vi "ReadProjectFromController_Example.vi"(8 "Fehler (Eingang, kein Fehler)":errorcluster, 11 "ControllerIP":string="192.168.5.24") -> (0 "Fehler (Ausgang)":errorcluster, 3 "ControllerID":string)   [LabVIEW 2016]
uses:
  girpcutil_params.ctl
panel:
  out "ConnectionToken":string
  out "ProjectPath":string
  out "ProjectID":string
  out "State":string
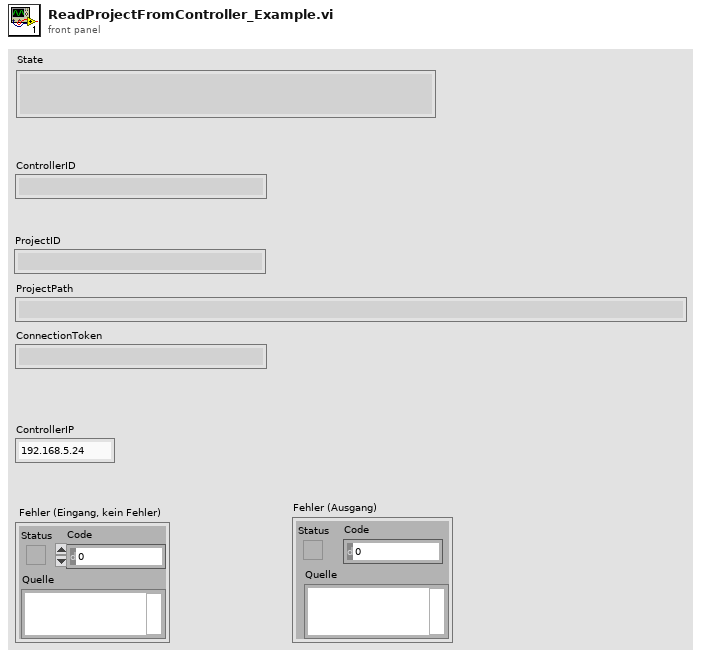
[diagram p1: front panel]
types:
  T1 = typedef "girpcutil_params.ctl" = cluster{"ConnectionHandle":i32, "DLL-Handle":cluster{"DLL Path":path, "Is32Bit":bool}}
  T2 = enum16{"Bool", "Snippet", "Struct", "Int64", "Int32", "Float", "Double", "String"}
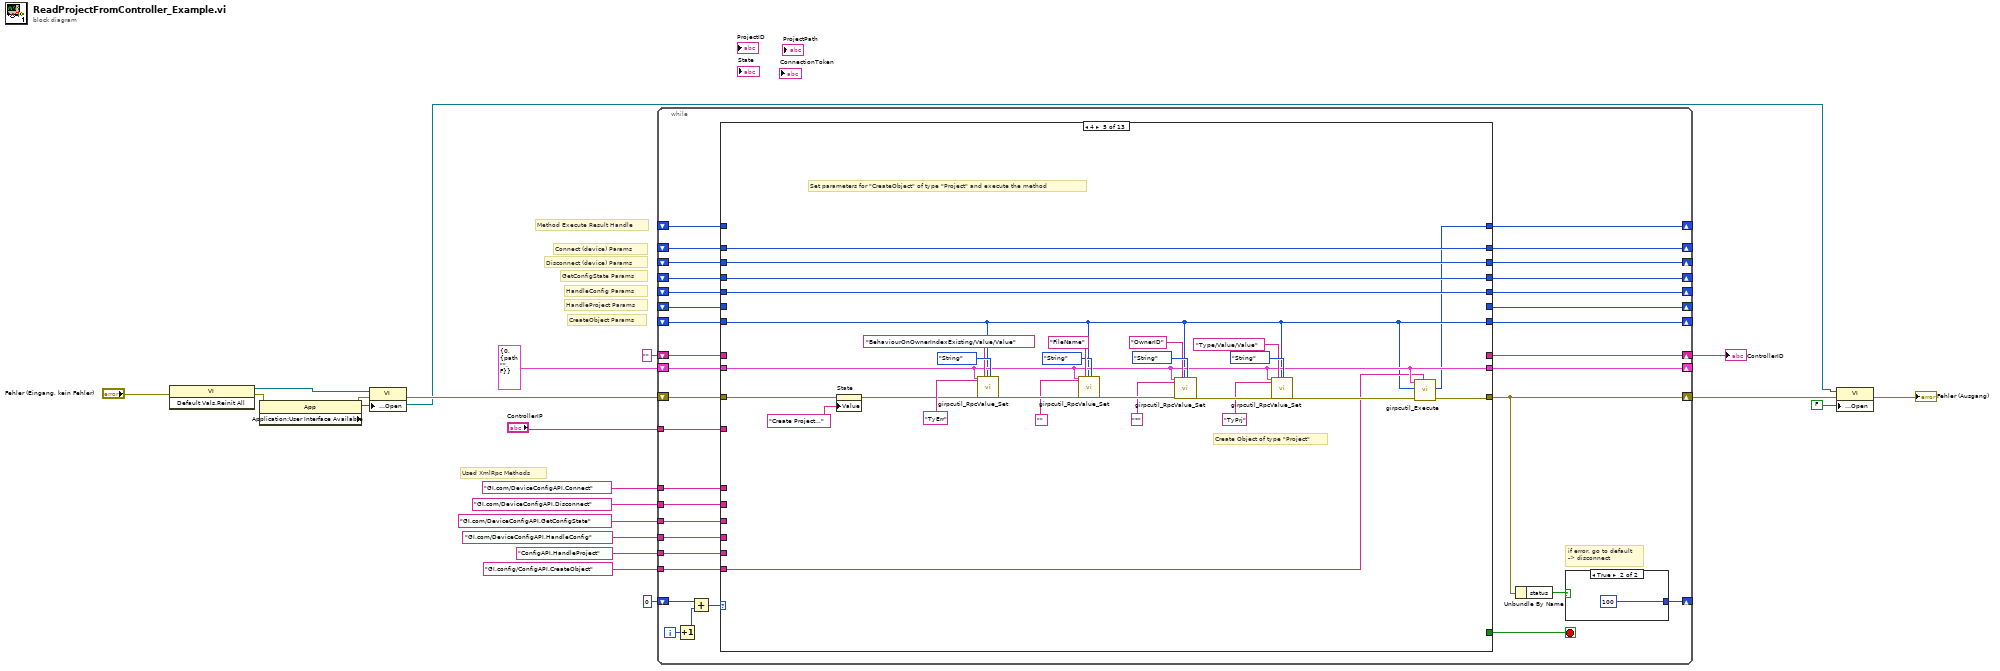
[diagram p0: block diagram]
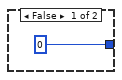
[diagram p2: hidden frame]
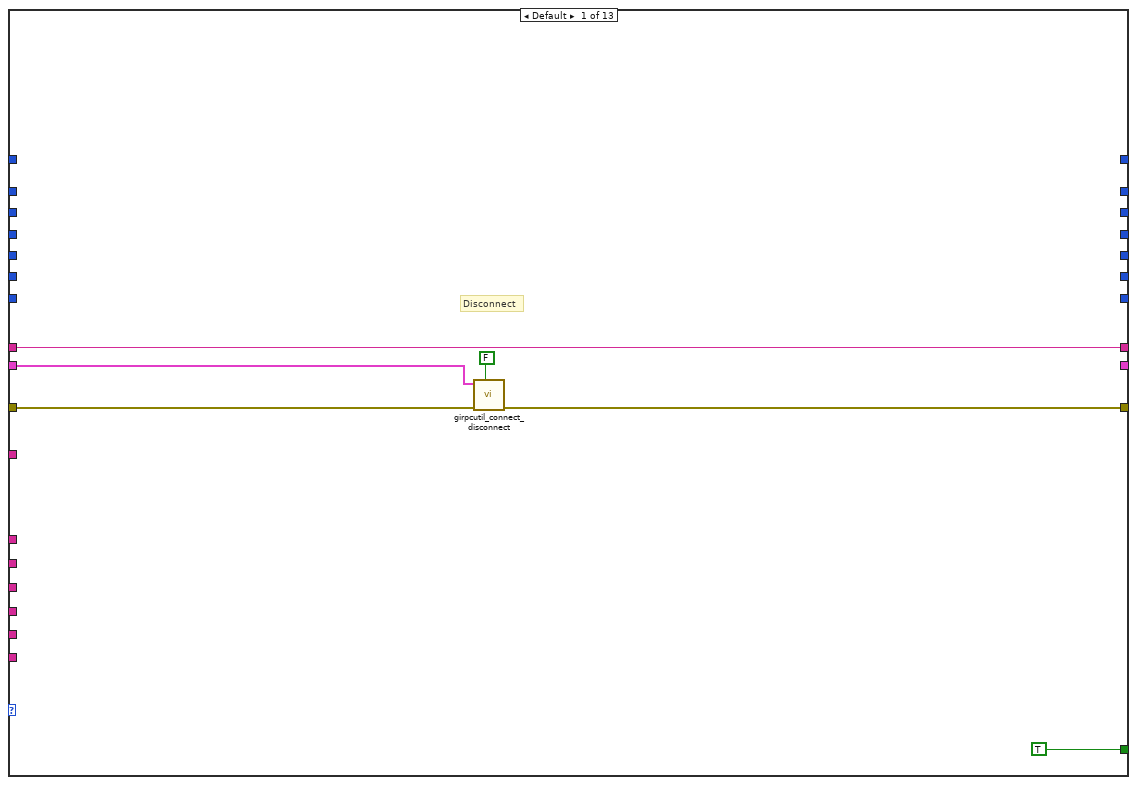
[diagram p3: hidden frame]
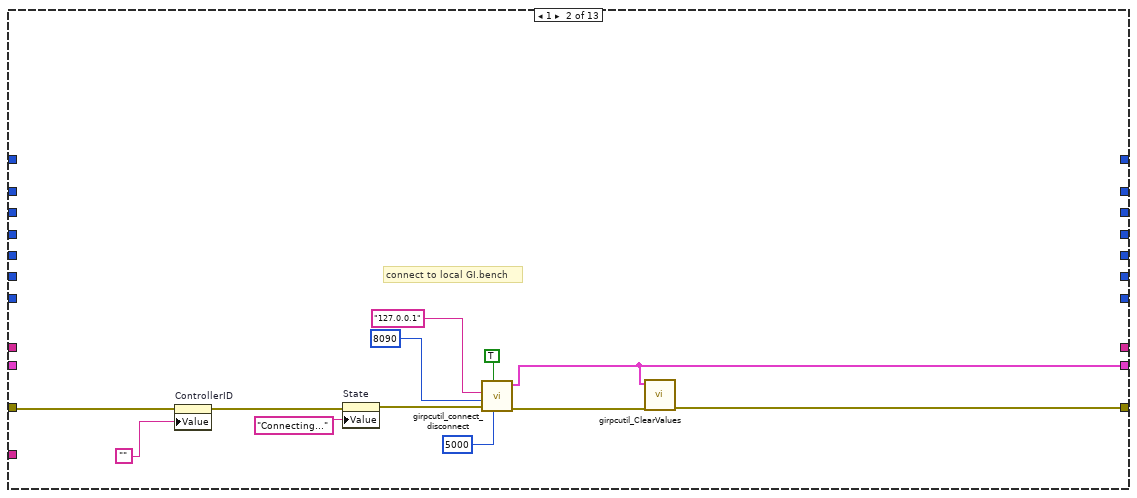
[diagram p4: hidden frame]
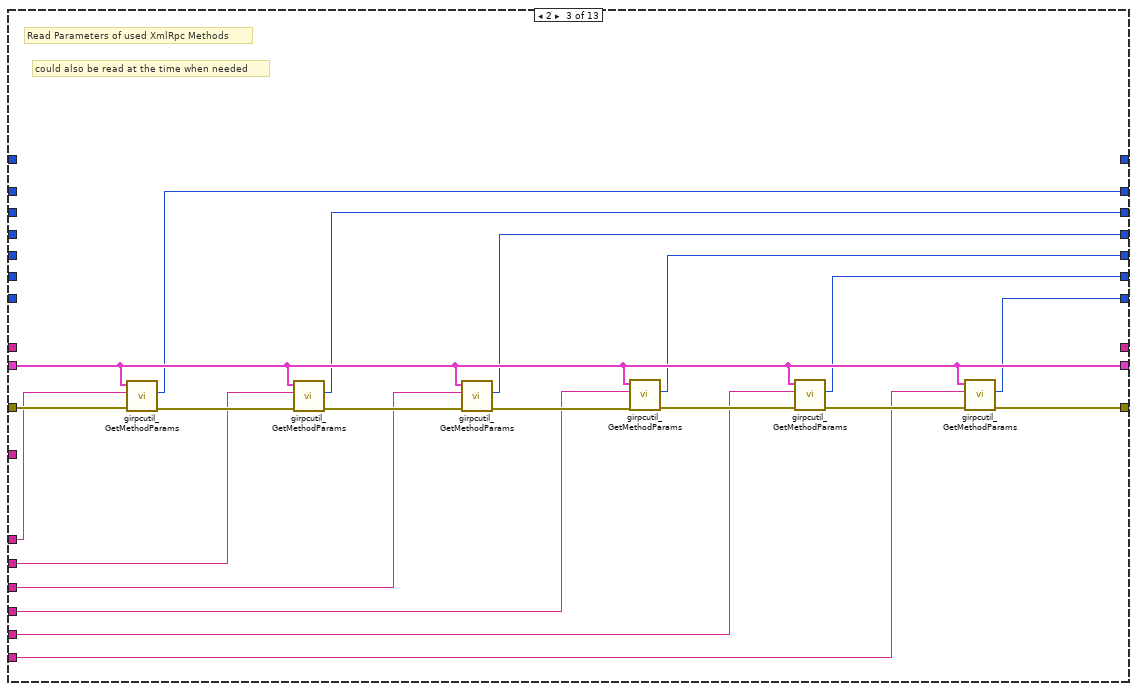
[diagram p5: hidden frame]
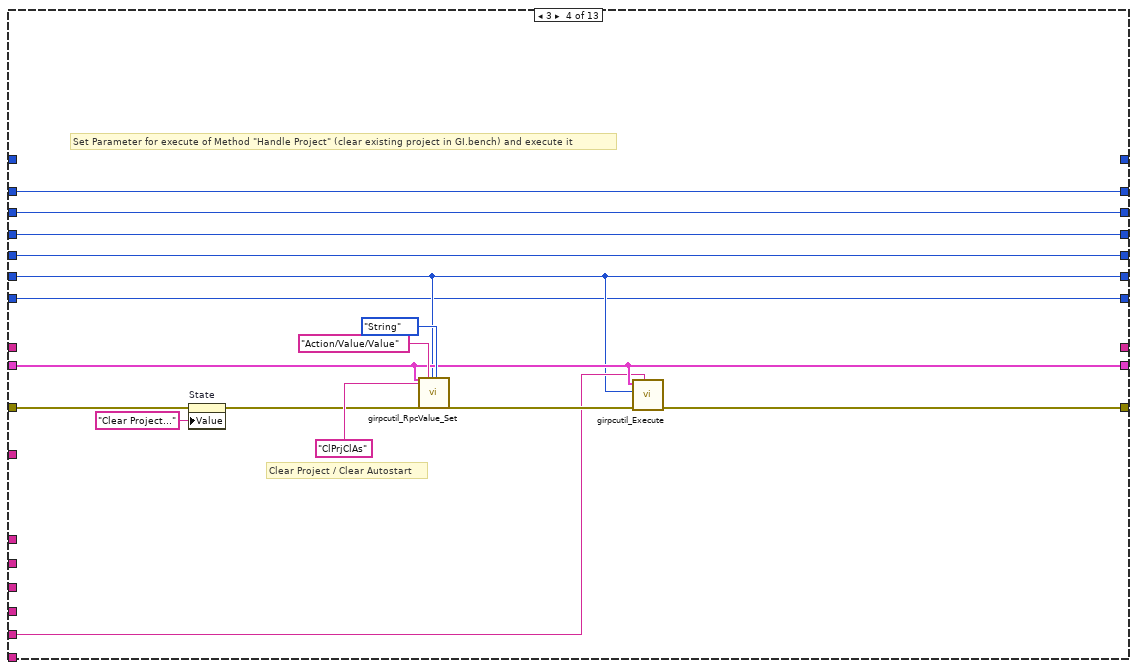
[diagram p6: hidden frame]
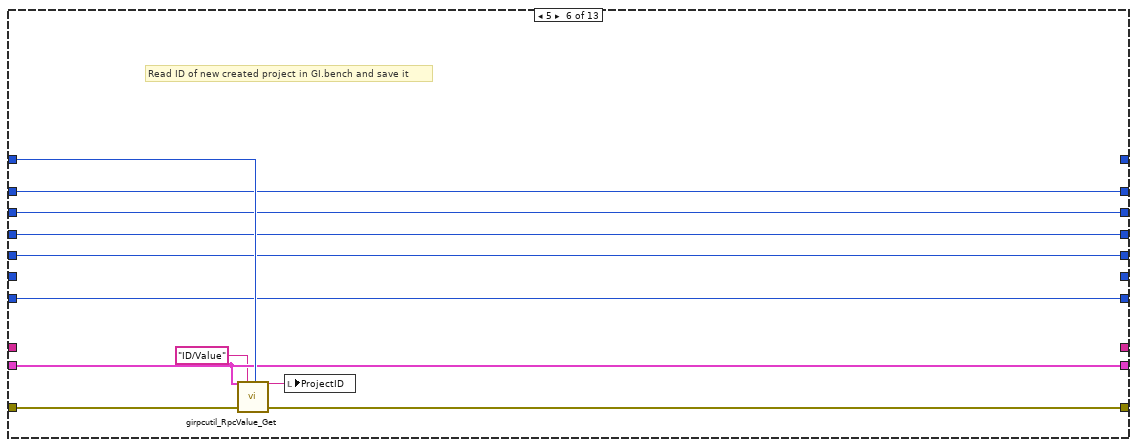
[diagram p7: hidden frame]
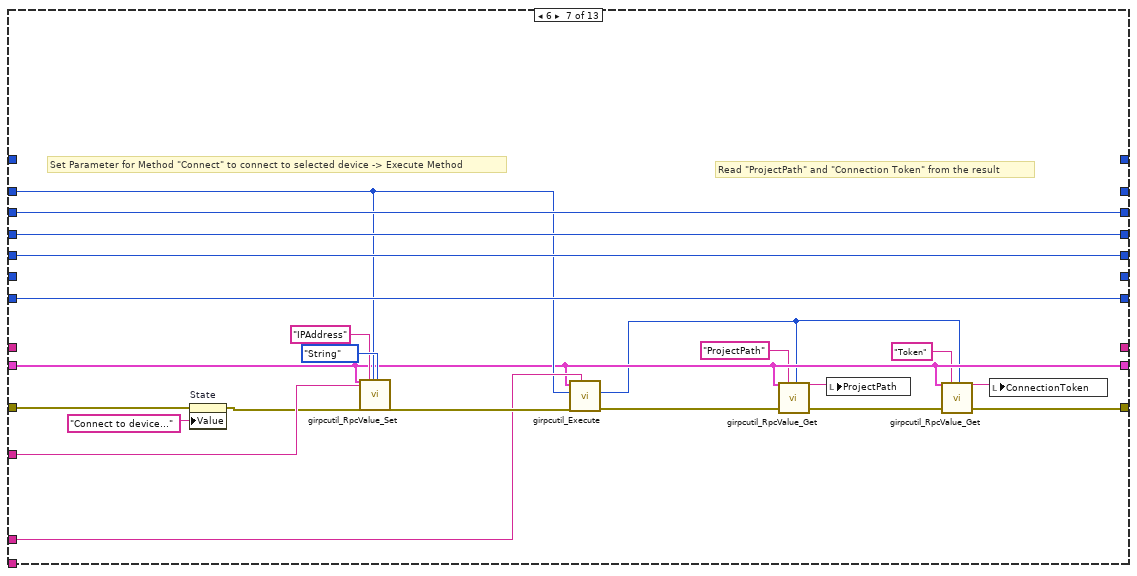
[diagram p8: hidden frame]
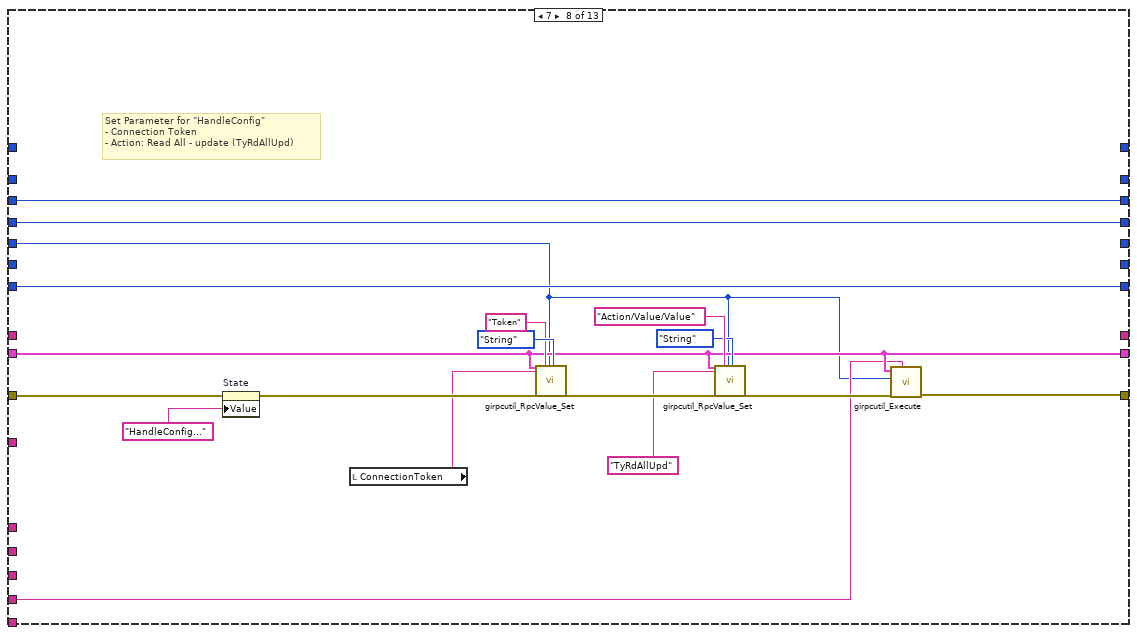
[diagram p9: hidden frame]
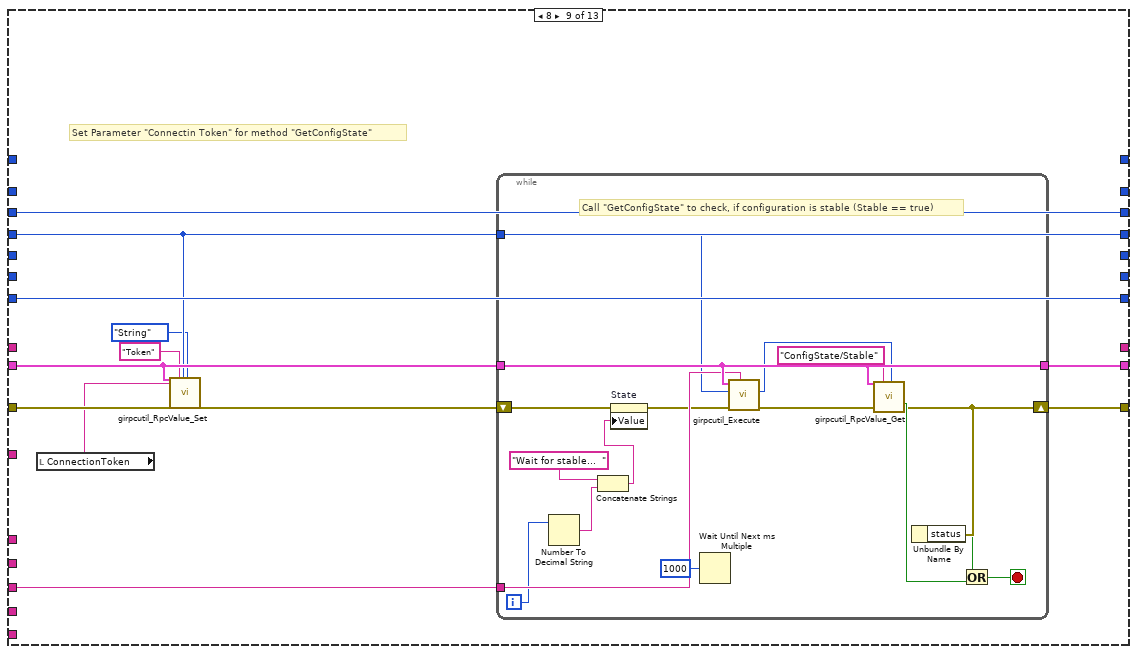
[diagram p10: hidden frame]
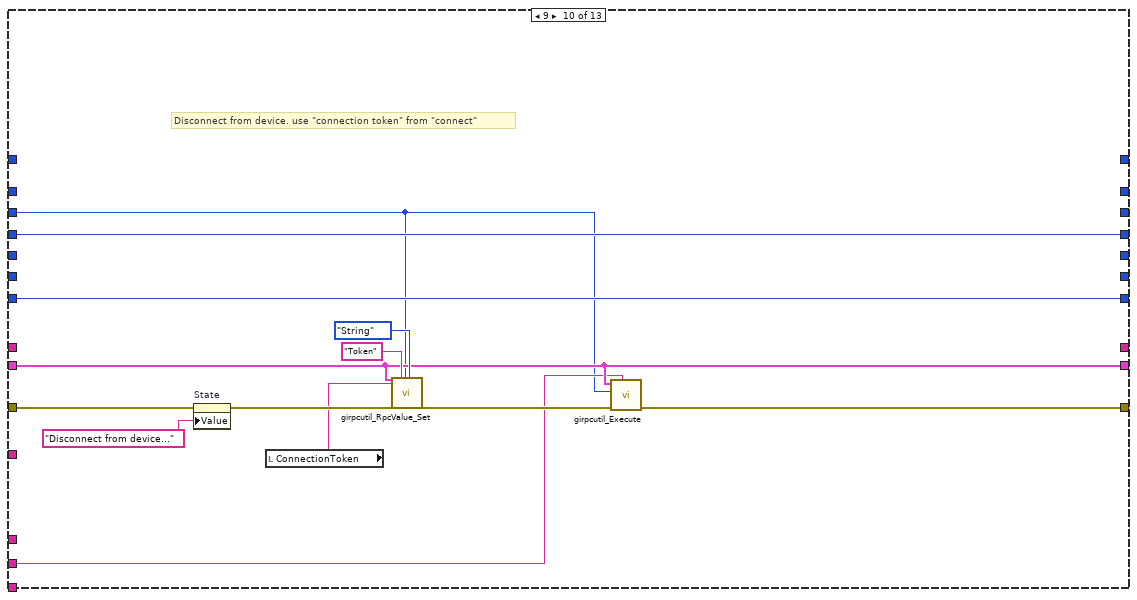
[diagram p11: hidden frame]
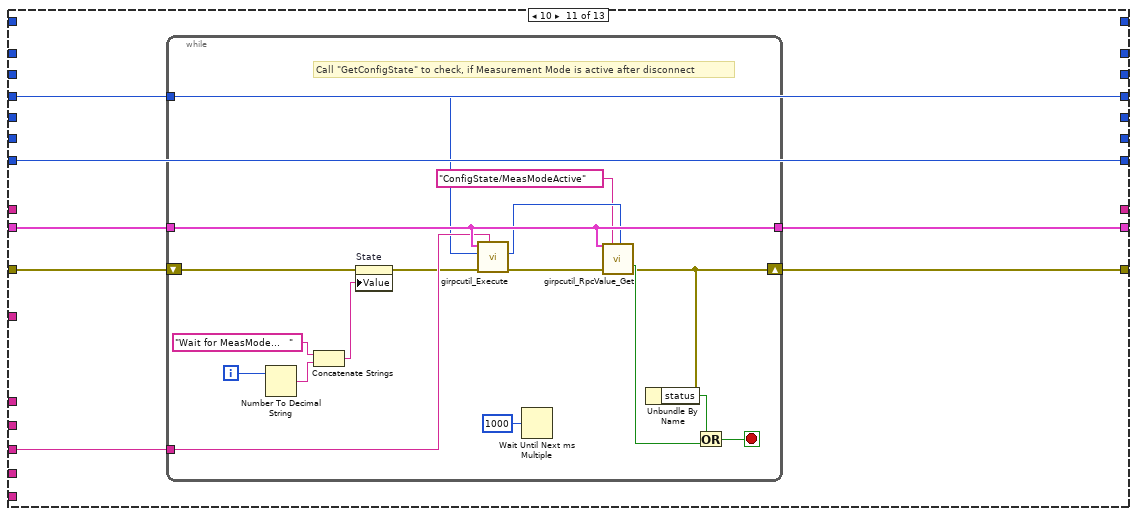
[diagram p12: hidden frame]
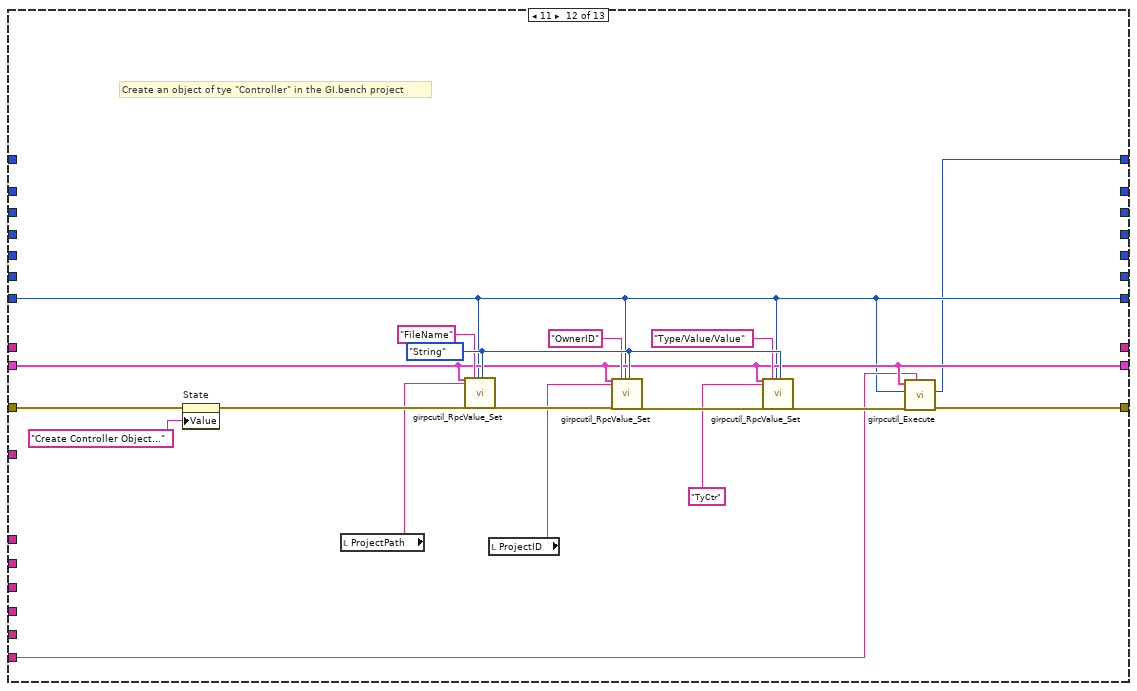
[diagram p13: hidden frame]
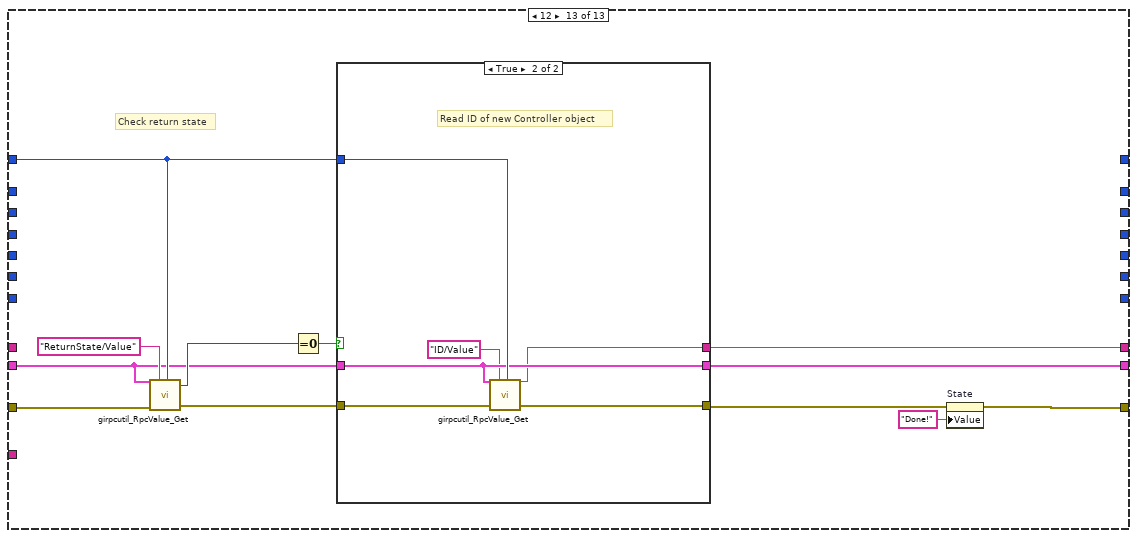
[diagram p14: hidden frame]
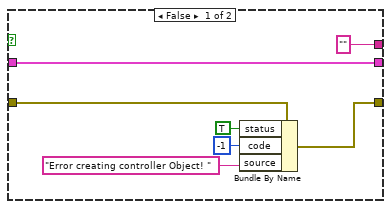
[diagram p15: hidden frame]
diagram:
  # "Method Execute Result Handle"
  # "CreateObject Params"
  # "HandleProject Params"
  # "HandleConfig Params"
  # "GetConfigState Params"
  # "Disconnect (device) Params"
  # "Connect (device) Params"
  # "Used XmlRpc Methods"
  n1 = invoke class="VI" method="Default Vals.Reinit All"(error in="Fehler (Eingang, kein Fehler)") -> (reference out=w13:refnum<vi>, error out=w11:errorcluster)  [unwired: 2 in, 1 out]
  n2 = property class="App"(error in=w11) -> (error out=w10:errorcluster, "Application:User Interface Available"=w12:bool)  [unwired: 1 in, 1 out]
  n3 = property class="VI"(reference=w13, error in=w10, "Front Panel.Open"=w12) -> (reference out=w4:refnum<vi>, error out=w9:errorcluster)
  n4 = while {
    shift-right: [w39] -> w6
    shift-left: w9 -> [w54]
    tunnel: "GI.com/DeviceConfigAPI.Connect" ("methodName") -> [w53]
    tunnel: "GI.com/DeviceConfigAPI.Disconnect" ("methodName") -> [w52]
    tunnel: "GI.com/DeviceConfigAPI.GetConfigState" ("methodName") -> [w51]
    tunnel: "GI.com/DeviceConfigAPI.HandleConfig" ("methodName") -> [w50]
    tunnel: "ConfigAPI.HandleProject" ("methodName") -> [w49]
    tunnel: "GI.config/ConfigAPI.CreateObject" ("methodName") -> [w48]
    shift-right: [w47] -> _
    shift-left: T1 {"ConnectionHandle"=0, "DLL-Handle"={"DLL Path"=path "", "Is32Bit"=FALSE}} ("girpcutil_params 2") -> [w46]
    shift-right: [w45] -> _
    shift-left: _ -> [w37]
    shift-right: [w44] -> _
    shift-left: _ -> [w36]
    shift-right: [w43] -> _
    shift-left: _ -> [w35]
    shift-right: [w42] -> _
    shift-left: _ -> [w34]
    shift-right: [w41] -> _
    shift-left: _ -> [w38]
    shift-right: [w40] -> _
    shift-left: _ -> [w33]
    shift-right: [w32] -> _
    shift-left: _ -> [w31]
    tunnel: "ControllerIP" -> [w30]
    shift-right: [w29] -> w15
    shift-left: "" ("StringResult") -> [w28]
    shift-right: [w22] -> _
    shift-left: 0 -> [w23]
    i -> [w55]
    stop <- w27 stop-if-true
    # "if error, go to default\n-> disconnect"
    n5 = Increment(x=w55) -> (x+1=w25:i32)
    n6 = Add(x=w23, y=w25) -> (x+y=w24:i32)
    n7 = case shown="4" w24 {
      tunnel: [TRUE _ _ _ _ _ _ _ _ _ _ _ _] -> w27
      tunnel: w54 -> [w62 w66 w95 w97 w113 w150 w154 w175 w197 w222 w239 w260 w286]
      tunnel: [w61 w70 w89 w107 w116 w146 w160 w177 w200 w227 w238 w266 w275] -> w39
      tunnel: w53 -> [_ _ w87 _ _ _ w164 _ _ _ _ _ _]
      tunnel: w52 -> [_ _ w86 _ _ _ _ _ _ w228 _ _ _]
      tunnel: w51 -> [_ _ w85 _ _ _ _ _ w201 _ w233 _ _]
      tunnel: w50 -> [_ _ w84 _ _ _ _ w179 _ _ _ _ _]
      tunnel: w49 -> [_ _ w83 w105 _ _ _ _ _ _ _ _ _]
      tunnel: w48 -> [_ _ w82 _ w118 _ _ _ _ _ _ w264 _]
      tunnel: [_ w69 w88 w106 w119 w148 w159 w180 w202 w229 w236 w265 w280] -> w47
      tunnel: w46 -> [w60 _ w88 w106 w119 w148 w159 w180 w195 w229 w237 w265 w279]
      tunnel: [_ _ w81 w103 w139 w145 _ _ _ _ _ _ _] -> w45
      tunnel: [_ _ w80 w102 w138 w144 w172 w188 w199 _ _ _ _] -> w44
      tunnel: [_ _ w79 w101 w137 w143 w171 w187 w194 w225 w235 _ _] -> w43
      tunnel: [_ _ w78 w100 w136 w142 w170 _ _ _ _ _ _] -> w42
      tunnel: [_ _ w77 w104 _ _ _ _ _ _ _ _ _] -> w41
      tunnel: [_ _ w76 w99 w117 w141 w169 w186 w198 w226 w234 w263 _] -> w40
      tunnel: w38 -> [_ _ _ w104 _ _ _ _ _ _ _ _ _]
      tunnel: w37 -> [_ _ _ w103 w139 w145 w163 _ _ _ _ _ _]
      tunnel: w36 -> [_ _ _ w102 w138 w144 w172 w188 w199 w224 _ _ _]
      tunnel: w35 -> [_ _ _ w101 w137 w143 w171 w187 w194 w225 w235 _ _]
      tunnel: w34 -> [_ _ _ w100 w136 w142 w170 w178 _ _ _ _ _]
      tunnel: w33 -> [_ _ _ w99 w117 w141 w169 w186 w198 w226 w234 w263 _]
      tunnel: [_ _ _ _ w115 _ _ _ _ _ _ w262 _] -> w32
      tunnel: w31 -> [_ _ _ _ _ w149 _ _ _ _ _ _ w281]
      tunnel: w30 -> [_ _ _ _ _ _ w166 _ _ _ _ _ _]
      tunnel: [w59 _ _ _ _ _ _ _ _ _ _ _ w278] -> w29
      tunnel: w28 -> [w59 _ _ _ _ _ _ _ _ _ _ _ _]
      frame Default {
        # "Disconnect"
        n8 = call "girpcutil_connect_disconnect.vi"("Connect"=FALSE, "Fehler (Eingang, kein Fehler)"=w62, "girpcutil_params"=w60) -> ("Fehler (Ausgang)"=w61:errorcluster)  [unwired: 7 in, 1 out]
      }
      frame 1 {
        # "connect to local GI.bench"
        n9 = property on="ControllerID" class="Str"(error in=w66, "Value"="") -> (error out=w65:errorcluster)  [unwired: 1 in, 1 out]
        n10 = property on="State" class="Str"(error in=w65, "Value"="Connecting..." ("State")) -> (error out=w68:errorcluster)  [unwired: 1 in, 1 out]
        n11 = call "girpcutil_connect_disconnect.vi"("timeout"=u32 5000, "Connect"=TRUE, "Fehler (Eingang, kein Fehler)"=w68, "port"=u32 8090, "host"="127.0.0.1") -> ("Fehler (Ausgang)"=w71:errorcluster, "girpcutil_params 2"=w69:T1)  [unwired: 5 in]
        n12 = call "girpcutil_ClearValues.vi"("Fehler (Eingang, kein Fehler)"=w71, "girpcutil_params"=w69) -> ("error IO"=w70:errorcluster)  [unwired: 9 in]
      }
      frame 2 {
        # "could also be read at the time when needed"
        # "Read Parameters of used XmlRpc Methods"
        n13 = call "girpcutil_GetMethodParams.vi"("Fehler (Eingang, kein Fehler)"=w95, "methodName"=w87, "girpcutil_params"=w88) -> ("Fehler (Ausgang)"=w94:errorcluster, "param handle out"=w81:i32)  [unwired: 7 in]
        n14 = call "girpcutil_GetMethodParams.vi"("Fehler (Eingang, kein Fehler)"=w94, "methodName"=w86, "girpcutil_params"=w88) -> ("Fehler (Ausgang)"=w93:errorcluster, "param handle out"=w80:i32)  [unwired: 7 in]
        n15 = call "girpcutil_GetMethodParams.vi"("Fehler (Eingang, kein Fehler)"=w93, "methodName"=w85, "girpcutil_params"=w88) -> ("Fehler (Ausgang)"=w92:errorcluster, "param handle out"=w79:i32)  [unwired: 7 in]
        n16 = call "girpcutil_GetMethodParams.vi"("Fehler (Eingang, kein Fehler)"=w92, "methodName"=w84, "girpcutil_params"=w88) -> ("Fehler (Ausgang)"=w91:errorcluster, "param handle out"=w78:i32)  [unwired: 7 in]
        n17 = call "girpcutil_GetMethodParams.vi"("Fehler (Eingang, kein Fehler)"=w91, "methodName"=w83, "girpcutil_params"=w88) -> ("Fehler (Ausgang)"=w90:errorcluster, "param handle out"=w77:i32)  [unwired: 7 in]
        n18 = call "girpcutil_GetMethodParams.vi"("Fehler (Eingang, kein Fehler)"=w90, "methodName"=w82, "girpcutil_params"=w88) -> ("Fehler (Ausgang)"=w89:errorcluster, "param handle out"=w76:i32)  [unwired: 7 in]
      }
      frame 3 {
        # "Clear Project / Clear Autostart"
        # "Set Parameter for execute of Method \"Handle Project\" (clear existing project in GI.bench) and execute it"
        n19 = property on="State" class="Str"(error in=w97, "Value"="Clear Project..." ("State")) -> (error out=w96:errorcluster)  [unwired: 1 in, 1 out]
        n20 = call "girpcutil_RpcValue_Set.vi"("girpcutil_params"=w106, "StringValue or Snippet"="ClPrjClAs", "Fehler (Eingang, kein Fehler)"=w96, "MemberName"="Action/Value/Value", "param handle"=w104, "DataType"=T2."String") -> ("Fehler (Ausgang)"=w108:errorcluster)  [unwired: 21 in]
        n21 = call "girpcutil_Execute.vi"("methodName"=w105, "Fehler (Eingang, kein Fehler)"=w108, "params"=w104, "girpcutil_params"=w106) -> ("Fehler (Ausgang)"=w107:errorcluster)  [unwired: 6 in, 1 out]
      }
      frame 4 {
        # "Create Object of type \"Project\""
        # "Set parameters for \"CreateObject\" of type \"Project\" and execute the method"
        n22 = property on="State" class="Str"(error in=w113, "Value"="Create Project..." ("State")) -> (error out=w112:errorcluster)  [unwired: 1 in, 1 out]
        n23 = call "girpcutil_RpcValue_Set.vi"("girpcutil_params"=w119, "StringValue or Snippet"="TyErr", "Fehler (Eingang, kein Fehler)"=w112, "MemberName"="BehaviourOnOwnerIndexExisting/Value/Value", "param handle"=w117, "DataType"=T2."String") -> ("Fehler (Ausgang)"=w132:errorcluster)  [unwired: 21 in]
        n24 = call "girpcutil_RpcValue_Set.vi"("girpcutil_params"=w119, "StringValue or Snippet"="", "Fehler (Eingang, kein Fehler)"=w132, "MemberName"="FileName", "param handle"=w117, "DataType"=T2."String") -> ("Fehler (Ausgang)"=w128:errorcluster)  [unwired: 21 in]
        n25 = call "girpcutil_RpcValue_Set.vi"("girpcutil_params"=w119, "StringValue or Snippet"="*", "Fehler (Eingang, kein Fehler)"=w128, "MemberName"="OwnerID", "param handle"=w117, "DataType"=T2."String") -> ("Fehler (Ausgang)"=w124:errorcluster)  [unwired: 21 in]
        n26 = call "girpcutil_RpcValue_Set.vi"("girpcutil_params"=w119, "StringValue or Snippet"="TyPrj", "Fehler (Eingang, kein Fehler)"=w124, "MemberName"="Type/Value/Value", "param handle"=w117, "DataType"=T2."String") -> ("Fehler (Ausgang)"=w120:errorcluster)  [unwired: 21 in]
        n27 = call "girpcutil_Execute.vi"("methodName"=w118, "Fehler (Eingang, kein Fehler)"=w120, "params"=w117, "girpcutil_params"=w119) -> ("Fehler (Ausgang)"=w116:errorcluster, "results"=w115:i32)  [unwired: 6 in]
      }
      frame 5 {
        # "Read ID of new created project in GI.bench and save it"
        n28 = call "girpcutil_RpcValue_Get.vi"("girpcutil_params"=w148, "Fehler (Eingang, kein Fehler)"=w150, "member"="ID/Value", "value"=w149) -> ("StringResult"=w140:string, "Fehler (Ausgang)"=w146:errorcluster)  [unwired: 19 in, 3 out]
        n29 = local write "ProjectID"(w140) -> ()
      }
      frame 6 {
        # "Read \"ProjectPath\" and \"Connection Token\" from the result"
        # "Set Parameter for Method \"Connect\" to connect to selected device -> Execute Method"
        n30 = property on="State" class="Str"(error in=w154, "Value"="Connect to device..." ("State")) -> (error out=w153:errorcluster)  [unwired: 1 in, 1 out]
        n31 = call "girpcutil_RpcValue_Set.vi"("girpcutil_params"=w159, "StringValue or Snippet"=w166, "Fehler (Eingang, kein Fehler)"=w153, "MemberName"="IPAddress", "param handle"=w163, "DataType"=T2."String") -> ("Fehler (Ausgang)"=w165:errorcluster)  [unwired: 21 in]
        n32 = call "girpcutil_Execute.vi"("methodName"=w164, "Fehler (Eingang, kein Fehler)"=w165, "params"=w163, "girpcutil_params"=w159) -> ("Fehler (Ausgang)"=w161:errorcluster, "results"=w158:i32)  [unwired: 6 in]
        n33 = call "girpcutil_RpcValue_Get.vi"("girpcutil_params"=w159, "Fehler (Eingang, kein Fehler)"=w161, "member"="ProjectPath", "value"=w158) -> ("StringResult"=w152:string, "Fehler (Ausgang)"=w162:errorcluster)  [unwired: 19 in, 3 out]
        n34 = local write "ProjectPath"(w152) -> ()
        n35 = call "girpcutil_RpcValue_Get.vi"("girpcutil_params"=w159, "Fehler (Eingang, kein Fehler)"=w162, "member"="Token", "value"=w158) -> ("StringResult"=w151:string, "Fehler (Ausgang)"=w160:errorcluster)  [unwired: 19 in, 3 out]
        n36 = local write "ConnectionToken"(w151) -> ()
      }
      frame 7 {
        # "Set Parameter for \"HandleConfig\"\n- Connection Token\n- Action: Read All - update (TyRdAllUpd)"
        n37 = property on="State" class="Str"(error in=w175, "Value"="HandleConfig..." ("State")) -> (error out=w174:errorcluster)  [unwired: 1 in, 1 out]
        n38 = local read "ConnectionToken"() -> (w173:string)
        n39 = call "girpcutil_RpcValue_Set.vi"("girpcutil_params"=w180, "StringValue or Snippet"=w173, "Fehler (Eingang, kein Fehler)"=w174, "MemberName"="Token", "param handle"=w178, "DataType"=T2."String") -> ("Fehler (Ausgang)"=w185:errorcluster)  [unwired: 21 in]
        n40 = call "girpcutil_RpcValue_Set.vi"("girpcutil_params"=w180, "StringValue or Snippet"="TyRdAllUpd", "Fehler (Eingang, kein Fehler)"=w185, "MemberName"="Action/Value/Value", "param handle"=w178, "DataType"=T2."String") -> ("Fehler (Ausgang)"=w181:errorcluster)  [unwired: 21 in]
        n41 = call "girpcutil_Execute.vi"("methodName"=w179, "Fehler (Eingang, kein Fehler)"=w181, "params"=w178, "girpcutil_params"=w180) -> ("Fehler (Ausgang)"=w177:errorcluster)  [unwired: 6 in, 1 out]
      }
      frame 8 {
        # "Set Parameter \"Connectin Token\" for method \"GetConfigState\""
        n42 = local read "ConnectionToken"() -> (w191:string)
        n43 = call "girpcutil_RpcValue_Set.vi"("girpcutil_params"=w195, "StringValue or Snippet"=w191, "Fehler (Eingang, kein Fehler)"=w197, "MemberName"="Token", "param handle"=w194, "DataType"=T2."String") -> ("Fehler (Ausgang)"=w196:errorcluster)  [unwired: 21 in]
        n44 = while {
          shift-right: [w210] -> w200
          shift-left: w196 -> [w208]
          tunnel: w195 -> [w218]
          tunnel: [w218] -> w202
          tunnel: w201 -> [w217]
          tunnel: w194 -> [w216]
          i -> [w204]
          stop <- w212 stop-if-true
          # "Call \"GetConfigState\" to check, if configuration is stable (Stable == true)"
          n45 = Number To Decimal String(number=w204) -> (decimal integer string=w203:string)  [unwired: 1 in]
          n46 = Concatenate Strings("Wait for stable...  " ("State"), w203) -> (w205:string)
          n47 = property on="State" class="Str"(error in=w208, "Value"=w205) -> (error out=w207:errorcluster)  [unwired: 1 in, 1 out]
          n48 = Wait Until Next ms Multiple(millisecond multiple=u32 1000) -> ()  [unwired: 1 out]
          n49 = call "girpcutil_Execute.vi"("methodName"=w217, "Fehler (Eingang, kein Fehler)"=w207, "params"=w216, "girpcutil_params"=w218) -> ("Fehler (Ausgang)"=w219:errorcluster, "results"=w215:i32)  [unwired: 6 in]
          n50 = call "girpcutil_RpcValue_Get.vi"("girpcutil_params"=w218, "Fehler (Eingang, kein Fehler)"=w219, "member"="ConfigState/Stable", "value"=w215) -> ("BoolResult"=w211:bool, "Fehler (Ausgang)"=w210:errorcluster)  [unwired: 19 in, 3 out]
          n51 = Unbundle By Name(w210) -> ("status"=w209:bool)
          n52 = Or(x=w209, y=w211) -> (x .or. y?=w212:bool)
        }
      }
      frame 9 {
        # "Disconnect from device. use \"connection token\" from \"connect\""
        n53 = property on="State" class="Str"(error in=w222, "Value"="Disconnect from device..." ("State")) -> (error out=w221:errorcluster)  [unwired: 1 in, 1 out]
        n54 = local read "ConnectionToken"() -> (w220:string)
        n55 = call "girpcutil_RpcValue_Set.vi"("girpcutil_params"=w229, "StringValue or Snippet"=w220, "Fehler (Eingang, kein Fehler)"=w221, "MemberName"="Token", "param handle"=w224, "DataType"=T2."String") -> ("Fehler (Ausgang)"=w230:errorcluster)  [unwired: 21 in]
        n56 = call "girpcutil_Execute.vi"("methodName"=w228, "Fehler (Eingang, kein Fehler)"=w230, "params"=w224, "girpcutil_params"=w229) -> ("Fehler (Ausgang)"=w227:errorcluster)  [unwired: 6 in, 1 out]
      }
      frame 10 {
        n57 = while {
          shift-right: [w247] -> w238
          shift-left: w239 -> [w245]
          tunnel: w237 -> [w255]
          tunnel: [w255] -> w236
          tunnel: w233 -> [w254]
          tunnel: w235 -> [w253]
          i -> [w240]
          stop <- w249 stop-if-true
          # "Call \"GetConfigState\" to check, if Measurement Mode is active after disconnect"
          n58 = Number To Decimal String(number=w240) -> (decimal integer string=w241:string)  [unwired: 1 in]
          n59 = Concatenate Strings("Wait for MeasMode...   " ("State"), w241) -> (w242:string)
          n60 = property on="State" class="Str"(error in=w245, "Value"=w242) -> (error out=w244:errorcluster)  [unwired: 1 in, 1 out]
          n61 = call "girpcutil_Execute.vi"("methodName"=w254, "Fehler (Eingang, kein Fehler)"=w244, "params"=w253, "girpcutil_params"=w255) -> ("Fehler (Ausgang)"=w256:errorcluster, "results"=w252:i32)  [unwired: 6 in]
          n62 = Wait Until Next ms Multiple(millisecond multiple=u32 1000) -> ()  [unwired: 1 out]
          n63 = call "girpcutil_RpcValue_Get.vi"("girpcutil_params"=w255, "Fehler (Eingang, kein Fehler)"=w256, "member"="ConfigState/MeasModeActive", "value"=w252) -> ("BoolResult"=w248:bool, "Fehler (Ausgang)"=w247:errorcluster)  [unwired: 19 in, 3 out]
          n64 = Unbundle By Name(w247) -> ("status"=w246:bool)
          n65 = Or(x=w246, y=w248) -> (x .or. y?=w249:bool)
        }
      }
      frame 11 {
        w272 = T2."String" ("DataType")
        # "Create an object of tye \"Controller\" in the GI.bench project"
        n66 = property on="State" class="Str"(error in=w260, "Value"="Create Controller Object..." ("State")) -> (error out=w259:errorcluster)  [unwired: 1 in, 1 out]
        n67 = local read "ProjectPath"() -> (w257:string)
        n68 = call "girpcutil_RpcValue_Set.vi"("girpcutil_params"=w265, "StringValue or Snippet"=w257, "Fehler (Eingang, kein Fehler)"=w259, "MemberName"="FileName", "param handle"=w263, "DataType"=w272) -> ("Fehler (Ausgang)"=w274:errorcluster)  [unwired: 21 in]
        n69 = local read "ProjectID"() -> (w258:string)
        n70 = call "girpcutil_RpcValue_Set.vi"("girpcutil_params"=w265, "StringValue or Snippet"=w258, "Fehler (Eingang, kein Fehler)"=w274, "MemberName"="OwnerID", "param handle"=w263, "DataType"=w272) -> ("Fehler (Ausgang)"=w273:errorcluster)  [unwired: 21 in]
        n71 = call "girpcutil_RpcValue_Set.vi"("girpcutil_params"=w265, "StringValue or Snippet"="TyCtr", "Fehler (Eingang, kein Fehler)"=w273, "MemberName"="Type/Value/Value", "param handle"=w263, "DataType"=w272) -> ("Fehler (Ausgang)"=w267:errorcluster)  [unwired: 21 in]
        n72 = call "girpcutil_Execute.vi"("methodName"=w264, "Fehler (Eingang, kein Fehler)"=w267, "params"=w263, "girpcutil_params"=w265) -> ("Fehler (Ausgang)"=w266:errorcluster, "results"=w262:i32)  [unwired: 6 in]
      }
      frame 12 {
        # "Check return state"
        n73 = call "girpcutil_RpcValue_Get.vi"("girpcutil_params"=w279, "Fehler (Eingang, kein Fehler)"=w286, "member"="ReturnState/Value", "value"=w281) -> ("Int64Result"=w283:i64, "Fehler (Ausgang)"=w282:errorcluster)  [unwired: 19 in, 3 out]
        n74 = Equal To 0?(x=w283) -> (x = 0?=w284:bool)
        n75 = case shown="True" w284 {
          tunnel: w282 -> [w289 w299]
          tunnel: w281 -> [_ w298]
          tunnel: [w292 w297] -> w280
          tunnel: w279 -> [w292 w297]
          tunnel: [w288 w295] -> w276
          tunnel: ["" ("StringResult") w294] -> w278
          frame False {
            n76 = Bundle By Name(cluster=w289, "status"=TRUE, "code"=-1, "source"="Error creating controller Object! ") -> (w288:errorcluster)
          }
          frame True {
            # "Read ID of new Controller object"
            n77 = call "girpcutil_RpcValue_Get.vi"("girpcutil_params"=w297, "Fehler (Eingang, kein Fehler)"=w299, "member"="ID/Value", "value"=w298) -> ("StringResult"=w294:string, "Fehler (Ausgang)"=w295:errorcluster)  [unwired: 19 in, 3 out]
          }
        }
        n78 = property on="State" class="Str"(error in=w276, "Value"="Done!" ("State")) -> (error out=w275:errorcluster)  [unwired: 1 in, 1 out]
      }
    }
    n79 = Unbundle By Name(w39) -> ("status"=w26:bool)
    n80 = case shown="True" w26 {
      tunnel: [0 100] -> w22
      frame False {
      }
      frame True {
      }
    }
  }
  "ControllerID" <- w15
  n81 = property class="VI"(reference=w4, error in=w6, "Front Panel.Open"=FALSE ("Frontpanel-Fenster:Öffnen")) -> (error out=→"Fehler (Ausgang)":errorcluster)  [unwired: 1 out]
